vi "TestMatrixTimeFreeze.vi"() -> ()   [LabVIEW 2022 SP3]
panel:
  in  "stop":bool
  out "max value":dbl
  in  "index":i32
  out "Array":dbl[](array[numeric])
  out "Power":dbl
  out "Time (s)":dbl
  out "concatenated string":string
  out "Intensity Graph":dbl[][](graph)
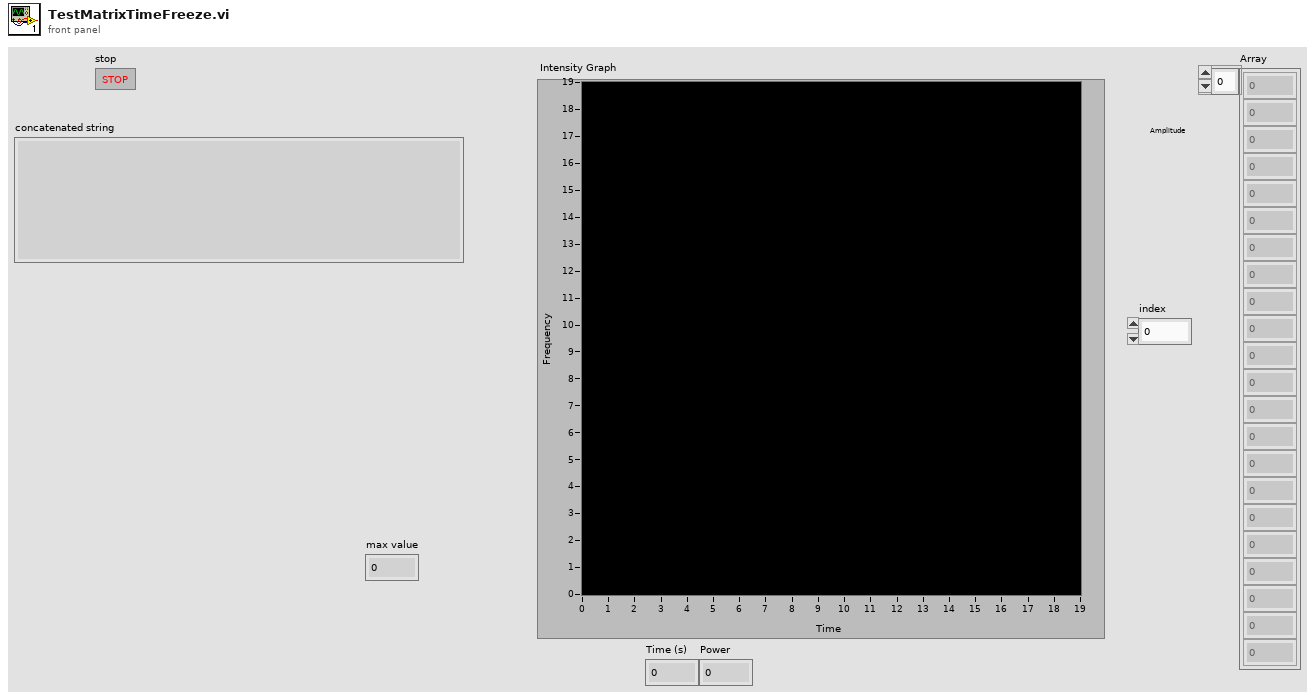
[diagram p1: front panel]
types:
  T1 = enum16{"open", "replace", "create", "open or create", "replace or create", "replace or create with confirmation"}
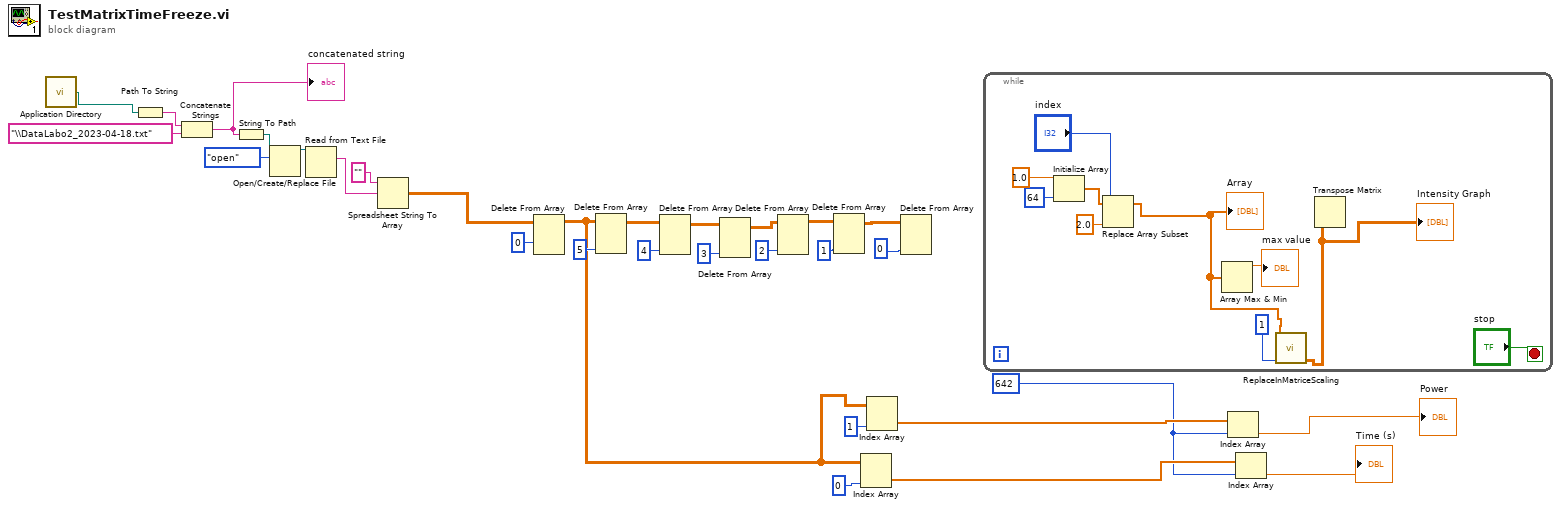
[diagram p0: block diagram]
diagram:
  w1 = 642
  n1 = call <vilib>:"Application Directory.vi"() -> ("Application Directory"=w11:path)
  n2 = Path To String(path=w11) -> (string=w30:string)
  n3 = Concatenate Strings(w30, "\\DataLabo2_2023-04-18.txt" ("string")) -> (w28:string)
  "concatenated string" <- w28
  n4 = String To Path(string=w28) -> (path=w27:path)
  n5 = Open/Create/Replace File(file path (use dialog)=w27, operation (0:open)=T1."open") -> (refnum out=w25:refnum<file>)  [unwired: 4 in, 2 out]
  n6 = Read from Text File(file (use dialog)=w25) -> (text=w24:string)  [unwired: 3 in, 3 out]
  n7 = Spreadsheet String To Array(format string="", spreadsheet string=w24) -> (array=w12:dbl[][])  [unwired: 2 in]
  n8 = Delete From Array(array=w12, index (row)=0) -> (array with subset deleted=w6:dbl[][])  [unwired: 2 in, 1 out]
  n9 = Delete From Array(array=w6, index (col)=5 ("disabled index (col)")) -> (array with subset deleted=w20:dbl[][])  [unwired: 2 in, 1 out]
  n10 = Delete From Array(array=w20, index (col)=4 ("disabled index (col)")) -> (array with subset deleted=w18:dbl[][])  [unwired: 2 in, 1 out]
  n11 = Delete From Array(array=w18, index (col)=3 ("disabled index (col)")) -> (array with subset deleted=w15:dbl[][])  [unwired: 2 in, 1 out]
  n12 = Delete From Array(array=w15, index (col)=2) -> (array with subset deleted=w14:dbl[][])  [unwired: 2 in, 1 out]
  n13 = Delete From Array(array=w14, index (col)=1 ("disabled index (col)")) -> (array with subset deleted=w9:dbl[][])  [unwired: 2 in, 1 out]
  n14 = Index Array(array=w6, index (col)=0 ("disabled index (col)")) -> (element=w2:dbl[])  [unwired: 1 in]
  n15 = Index Array(array=w6, index (col)=1) -> (element=w3:dbl[])  [unwired: 1 in]
  n16 = Delete From Array(array=w9, index (col)=0) -> ()  [unwired: 2 in, 2 out]
  n17 = while {
    stop <- "stop" stop-if-true
    n18 = Initialize Array(1.0 ("element"), 64 ("dimension size")) -> (w36:dbl[])
    n19 = Replace Array Subset(array=w36, new element=2.0 ("new element/subarray"), index="index") -> (w33:dbl[])
    "Array" <- w33
    n20 = Array Max & Min(array=w33) -> (max value=→"max value":dbl)  [unwired: 3 out]
    n21 = call "ReplaceInMatriceScaling.vi"("Input Scaling"=1, "Input Array"=w33) -> ("Output Array"=w38:dbl[][])  [unwired: 9 in]
    "Intensity Graph" <- w38
    n22 = Transpose Matrix(1:w38) -> ()  [unwired: 1 out]
  }
  n23 = Index Array(array=w3, index=w1) -> (element=→"Power":dbl)
  n24 = Index Array(array=w2, index=w1) -> (element=→"Time (s)":dbl)
